vi "GetIniPaths.vi"(7 "Severity":string, 8 "Error Array In":errorcluster[](array[cluster]), 10 "ModuleList":string[](array[string]), 11 "Test.lvclass":refnum<class "Test.lvclass">) -> (0 "Error Array Out":errorcluster[](array[cluster]), 2 "Script Locations":path[](array[path]), 3 "Test.lvclass":refnum<class "Test.lvclass">)   [LabVIEW 2018, in "Test.lvclass"]
doc: "Extracts the path to the ini configuration(s) file path based on the list of modules currently in use."
uses:
  Test.lvclass
  Test.lvclass/Test.ctl
  Accessors/Read ErrorSeverity.vi
  Accessors/Read PluginPathArray.vi
  Accessors/Read PluginIndex.vi
  <userlib>/NIST/NISTErrorLib/NISTErrorLib.lvlib
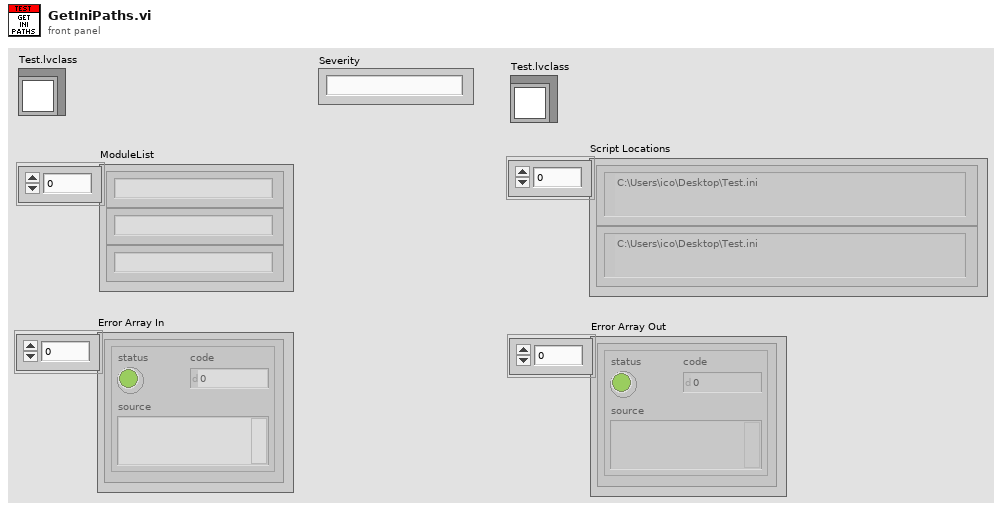
[diagram p1: front panel]
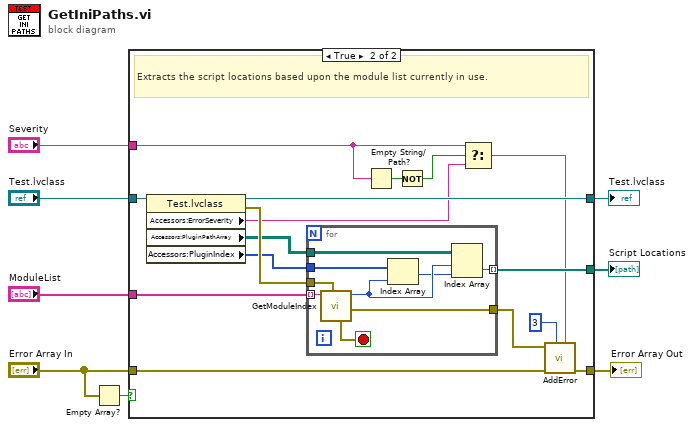
[diagram p0: block diagram]
diagram:
  n1 = Empty Array?(array="Error Array In") -> (empty?=w3:bool)
  n2 = case shown="True" w3 {
    tunnel: "Error Array In" -> [w9 w26]
    tunnel: [w9 w25] -> w2
    tunnel: "ModuleList" -> [_ w24]
    tunnel: "Test.lvclass" -> [w10 w23]
    tunnel: [_ w22] -> w6
    tunnel: [w10 w21] -> w5
    tunnel: "Severity" -> [_ w13]
    frame False {
    }
    frame True {
      # "Extracts the script locations based upon the module list currently in use."
      n3 = property class="Test.lvclass"(reference=w23) -> (reference out=w21:refnum<class "Test.lvclass">, error out=w20:errorcluster, "Accessors:ErrorSeverity"=w14:string, "Accessors:PluginPathArray"=w18:path[][], "Accessors:PluginIndex"=w19:u32[])  [unwired: 1 in]
      n4 = for {
        tunnel: w24 -> [w34] mode=indexing
        tunnel: w20 -> [w33]
        tunnel: w19 -> [w32]
        tunnel: w18 -> [w31]
        tunnel: [w28] -> w22 mode=indexing
        tunnel: [w27] -> w17
        stop <- w27 stop-if-true
        n5 = call "GetModuleIndex.vi"("Error In"=w33, "ModuleType"=w34) -> ("ModuleIndex"=w30:i32, "Error"=w27:errorcluster)  [unwired: 8 in]
        n6 = Index Array(array=w32, index=w30) -> (element=w29:u32)
        n7 = Index Array(array=w31, index (row)=w30, index (col)=w29) -> (element=w28:path)
      }
      n8 = Empty String/Path?(string/path=w13) -> (empty?=w12:bool)
      n9 = Not(x=w12) -> (.not. x?=w11:bool)
      n10 = Select(t=w13, s=w11, f=w14) -> (s? t:f=w15:string)
      n11 = call <userlib>:"AddError.vi"("Severity"=w15, "Priority"=u8 3, "ErrorArray In"=w26, "error in (no error)"=w17) -> ("ErrorArray Out"=w25:errorcluster[])  [unwired: 6 in, 1 out]
    }
  }
  "Test.lvclass" <- w5
  "Script Locations" <- w6
  "Error Array Out" <- w2
